vi "Initialize Attributes Core.vi"(8 "error in (no error)":errorcluster, 10 "Attribute Data":variant, 11 "BNT_SLMsgLogger in":refnum<class "BNT_SLMsgLogger.lvclass">) -> (0 "error out":errorcluster, 2 "MandatoryParameters":cluster{"Parameter":string, "found?":bool}[](array[cluster]), 3 "BNT_SLMsgLogger out":refnum<class "BNT_SLMsgLogger.lvclass">)   [LabVIEW 2019, in "BNT_SLMsgLogger.lvlib" / "BNT_SLMsgLogger.lvclass"]
doc: "Initialize object attribute.\n\nUnique resources should be allocated elsewhere!"
uses:
  BNT_SLMsgLogger.lvclass
  Protocol.ctl
  BNT_SLMsgLogger.lvclass/BNT_SLMsgLogger.ctl
  <vilib>/Skyline/Configuration/Configuration AMQP_class/NI Skyline Configuration AMQP.lvclass
  C:/Program Files (x86)/National Instruments/LabVIEW 2019/vi.lib/Skyline/Configuration/Configuration_class/NI Skyline Configuration.lvclass
  <vilib>/Skyline/Configuration/Configuration HTTP_class/NI Skyline Configuration HTTP.lvclass
  CSPP_Core/Classes/CSPP_BaseClasses/MessageLogger/CSPP_MessageLogger.lvclass
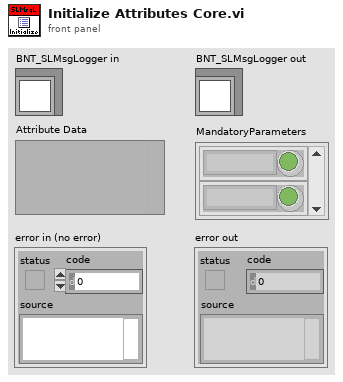
[diagram p1: front panel]
types:
  T1 = typedef "BNT_SLMsgLogger.lvlib/BNT_SLMsgLogger.lvclass/Protocol.ctl" = enum16{"AMQPSync", "AMQPAsync", "HTTP"}
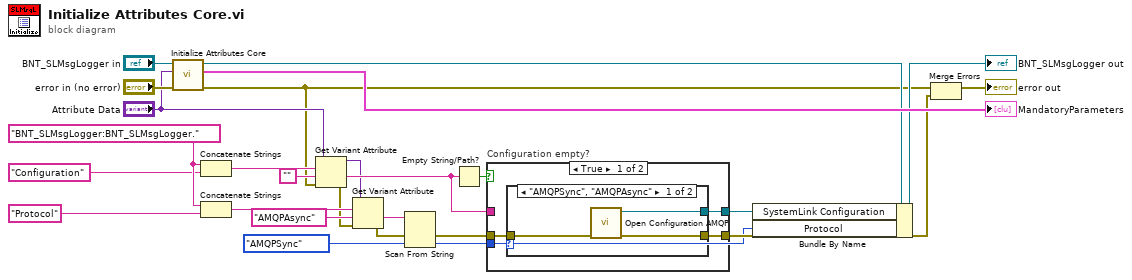
[diagram p0: block diagram]
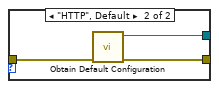
[diagram p2: hidden frame]
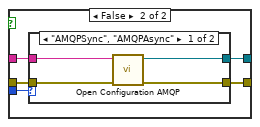
[diagram p3: hidden frame]
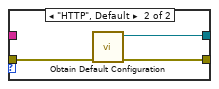
[diagram p4: hidden frame]
diagram:
  w10 = "BNT_SLMsgLogger:BNT_SLMsgLogger."
  n1 = call-parent "Initialize Attributes Core.vi"("error in (no error)"="error in (no error)", "Attribute Data"="Attribute Data", "CSPP_Base in"="BNT_SLMsgLogger in") -> ("error out"=w3:errorcluster, "MandatoryParameters"=→"MandatoryParameters":cluster{"Parameter":string, "found?":bool}[], "CSPP_Base out"=w23:refnum<class "BNT_SLMsgLogger.lvclass">)  [unwired: 6 in]
  n2 = Concatenate Strings(w10, "Configuration") -> (w8:string)
  n3 = Concatenate Strings(w10, "Protocol") -> (w19:string)
  n4 = Get Variant Attribute(Variant="Attribute Data", name=w8, default value (empty Variant)="", error in=w3) -> (duplicate Variant=w2:variant, value=w5:string, error out=w1:errorcluster)  [unwired: 1 out]
  n5 = Get Variant Attribute(Variant=w2, name=w19, default value (empty Variant)="AMQPAsync", error in=w1) -> (value=w17:string, error out=w11:errorcluster)  [unwired: 2 out]
  n6 = Scan From String(input string=w17, error in=w11, default 1=Protocol."AMQPSync" ("Protocol")) -> (error out=w15:errorcluster, output 1=w12:T1)  [unwired: 2 in, 2 out]
  n7 = Empty String/Path?(string/path=w5) -> (empty?=w6:bool)
  n8 = case "Configuration empty?" shown="True" w6 {
    tunnel: [w30 w41] -> w21
    tunnel: w15 -> [w29 w40]
    tunnel: [w28 w39] -> w13
    tunnel: w12 -> [w27 w38]
    tunnel: w5 -> [_ w37]
    frame True {
      n9 = case shown="\"AMQPSync\", \"AMQPAsync\"" w27 {
        tunnel: [w31 w36] -> w30
        tunnel: w29 -> [w33 w35]
        tunnel: [w32 w34] -> w28
        frame "AMQPSync", "AMQPAsync" {
          n10 = call <vilib>:"Open Configuration AMQP.vi"("error in (no error)"=w33) -> ("error out"=w32:errorcluster, "configuration"=w31:refnum<class "NI Skyline Configuration AMQP.lvclass">)  [unwired: 9 in]
        }
        frame "HTTP", Default {
          n11 = call <vilib>:"Obtain Default Configuration.vi"("error in (no error)"=w35) -> ("error out"=w34:errorcluster, "HTTP configuration out"=w36:refnum<class "NI Skyline Configuration HTTP.lvclass">)  [unwired: 9 in]
        }
      }
    }
    frame False {
      n12 = case shown="\"AMQPSync\", \"AMQPAsync\"" w38 {
        tunnel: [w43 w48] -> w41
        tunnel: w40 -> [w45 w47]
        tunnel: [w44 w46] -> w39
        tunnel: w37 -> [w42 _]
        frame "AMQPSync", "AMQPAsync" {
          n13 = call <vilib>:"Open Configuration AMQP.vi"("error in (no error)"=w45, "configuration id"=w42) -> ("error out"=w44:errorcluster, "configuration"=w43:refnum<class "NI Skyline Configuration AMQP.lvclass">)  [unwired: 8 in]
        }
        frame "HTTP", Default {
          n14 = call <vilib>:"Obtain Default Configuration.vi"("error in (no error)"=w47) -> ("error out"=w46:errorcluster, "HTTP configuration out"=w48:refnum<class "NI Skyline Configuration HTTP.lvclass">)  [unwired: 9 in]
        }
      }
    }
  }
  n15 = Bundle By Name(cluster=w23, "SystemLink Configuration"=w21, "Protocol"=w12) -> (→"BNT_SLMsgLogger out":refnum<class "BNT_SLMsgLogger.lvclass">)
  n16 = Merge Errors(w3, w13) -> (→"error out":errorcluster)
